vi "GP22_TDC_Arduinoed Single Measurement.vi"() -> ()   [LabVIEW 2013, in "GP22_TDC_Arduinoed.lvlib"]
uses:
  GP22_TDC_Arduinoed.lvlib
panel:
  out "Calibration / s":dbl format="%^#_6g"
  out "output / s":dbl format="%^#_6g"
  out "Freq / Hz":dbl
  out "error out":errorcluster
  out "Self-Test Result Message":string
  in  "VISA resource name":refnum<visa-resource-name>
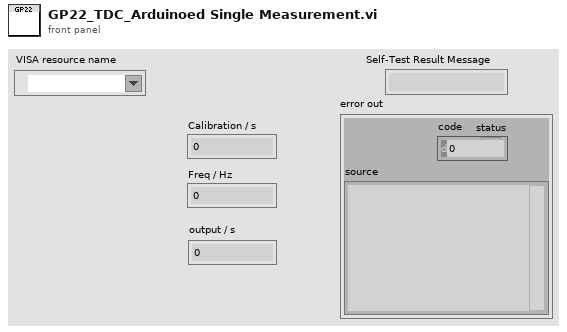
[diagram p1: front panel]
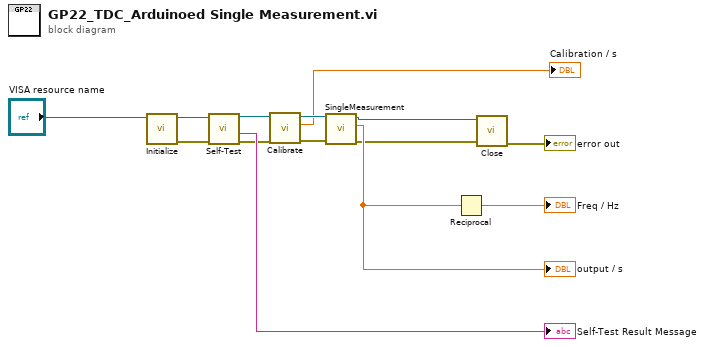
[diagram p0: block diagram]
diagram:
  n1 = call "Initialize.vi"("VISA resource name"="VISA resource name") -> ("error out"=w12:errorcluster, "VISA resource name out"=w13:refnum<visa-resource-name>)  [unwired: 9 in]
  n2 = call "Self-Test.vi"("error in (no error)"=w12, "VISA resource name"=w13) -> ("error out"=w4:errorcluster, "Self-Test Result Message"=→"Self-Test Result Message":string, "VISA resource name out"=w5:refnum<visa-resource-name>)  [unwired: 6 in, 1 out]
  n3 = call "Calibrate.vi"("error in (no error)"=w4, "VISA resource name"=w5) -> ("error out"=w3:errorcluster, "output / s"=→"Calibration / s":dbl, "VISA resource name out"=w6:refnum<visa-resource-name>)  [unwired: 5 in, 1 out]
  n4 = call "SingleMeasurement.vi"("error in (no error)"=w3, "VISA resource name"=w6) -> ("error out"=w2:errorcluster, "output / s"=w7:dbl, "VISA resource name out"=w9:refnum<visa-resource-name>)  [unwired: 7 in]
  "output / s" <- w7
  n5 = Reciprocal(x=w7) -> (1/x=→"Freq / Hz":dbl)
  n6 = call "Close.vi"("error in (no error)"=w2, "VISA resource name"=w9) -> ("error out"=→"error out":errorcluster)  [unwired: 9 in]
